vi "readAmountOfSelected.vi"(8 "error in (no error)":errorcluster, 11 "SingleSelectMCLBAdapter in":refnum<class "SingleSelectMCLBAdapter.lvclass">) -> (0 "error out":errorcluster, 2 "Numeric":dbl, 3 "SingleSelectMCLBAdapter out":refnum<class "SingleSelectMCLBAdapter.lvclass">)   [LabVIEW 2020, in "SingleSelectMCLBAdapter.lvclass"]
uses:
  SingleSelectMCLBAdapter.lvclass
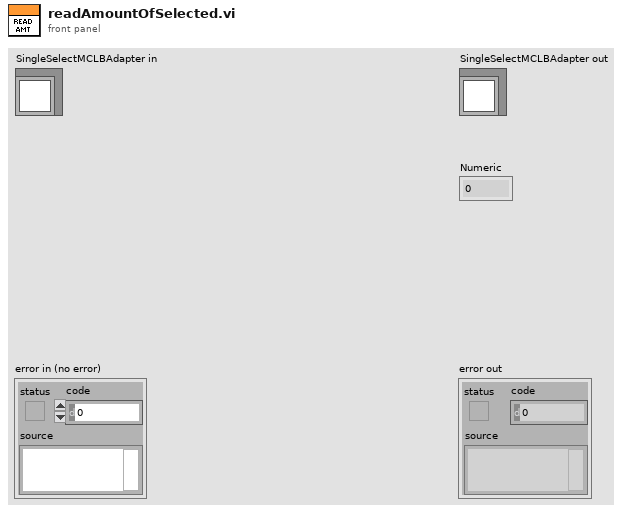
[diagram p1: front panel]
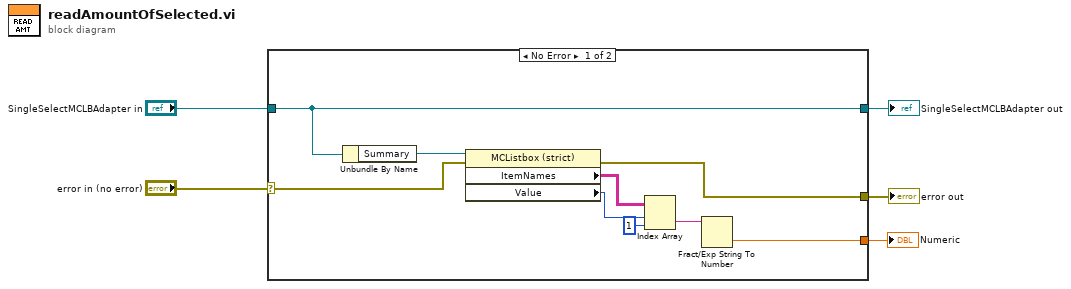
[diagram p0: block diagram]
diagram:
  n1 = case shown="No Error" "error in (no error)" {
    selector: "error in (no error)" -> [w9 w16]
    tunnel: [w8 w16] -> w4
    tunnel: [w10 w15] -> w2
    tunnel: "SingleSelectMCLBAdapter in" -> [w10 w15]
    tunnel: [w6 _] -> w1
    frame No Error {
      n2 = Unbundle By Name(w10) -> ("Summary"=w14:refnum<vi>)
      n3 = property class="MCListbox (strict)"(reference=w14, error in=w9) -> (error out=w8:errorcluster, "ItemNames"=w13:string[][], "Value"=w12:i32)  [unwired: 1 out]
      n4 = Index Array(array=w13, index (row)=w12, index (col)=1 ("disabled index (col)")) -> (element=w7:string)
      n5 = Fract/Exp String To Number(string=w7) -> (number=w6:dbl)  [unwired: 3 in, 1 out]
    }
    frame Error {
    }
  }
  "error out" <- w4
  "SingleSelectMCLBAdapter out" <- w2
  "Numeric" <- w1
